vi "createWriterQueue.vi"(0 "QueueName":string, 2 "WriterEndPointName":string, 5 "error in":errorcluster, 6 "ReaderEndPointName":string, 8 "Remote application Name":string) -> (19 "error out":errorcluster)   [LabVIEW 2013]
doc: "Used as a mechanism to have queue notification across process boundaries using network streams. No need to define a shared variable. Put the vi outside of the loop in parallel, and define a named queue to communicate through the link.\n\nRemote application Name - Remote application process instance name that tells the writer where to send the data \nReaderEndPointName - Used to build up the application context indicating the endpoint to stream data. Make sure that this matches both sides of the link.\nQueueName - Named queue to be used within the process.\nWriterEndPointName - Application process instance name that indicates where the data stream is sourced from"
uses:
  control/payloadData.ctl
  control/cmdQueueWriterRef.ctl
  Global/GlobalStop.vi
  <resource>/objmgr/ni.dex.rc
panel:
  out "Main Loop":i32
  out "writerURL":string
  out "Application:Name":string
  out "errorLoop":i32
  out "readerURL":string
  out "Acquire loop":i32
  out "queue OP":T1
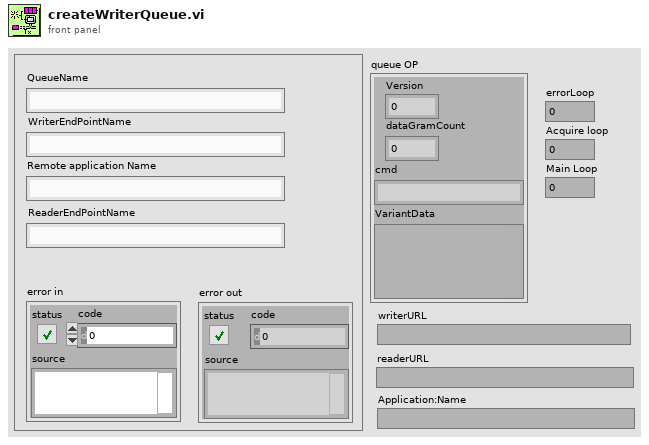
[diagram p1: front panel]
types:
  T1 = typedef "payloadData.ctl" = cluster{"Version":u32, "dataGramCount":i32, "cmd":string, "VariantData":variant}
  T2 = enum32{"invalid app kind", "Development System", "Run Time System", "Student Edition", "Embedded LabVIEW", "Evaluation", "Custom"}
  T3 = typedef "cmdQueueWriterRef.ctl" = cluster{"cmd":string, "msgQueue":refnum<queue>, "writerEndPoint":refnum<k21>}
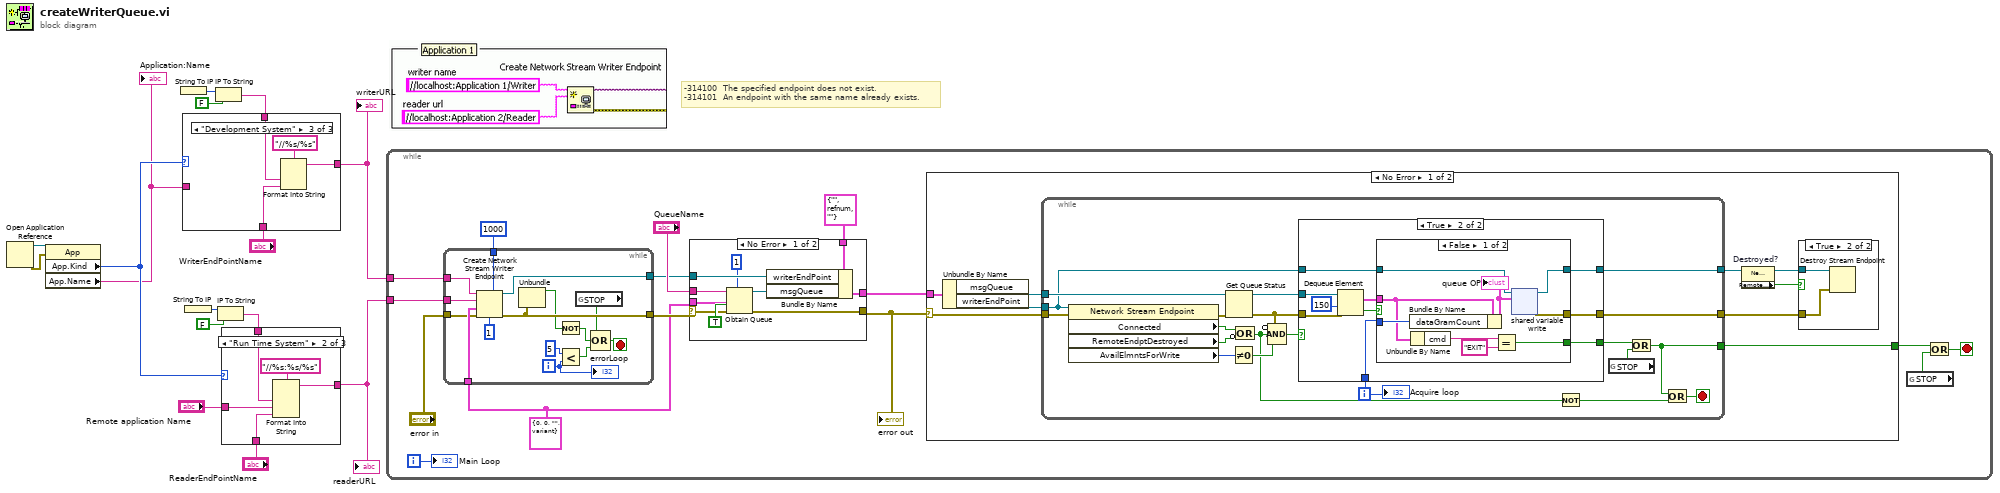
[diagram p0: block diagram]
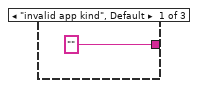
[diagram p2: hidden frame]
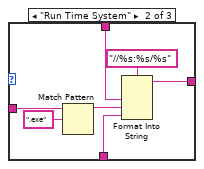
[diagram p3: hidden frame]
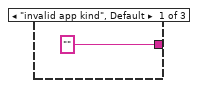
[diagram p4: hidden frame]
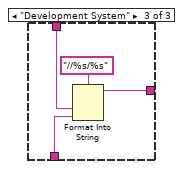
[diagram p5: hidden frame]
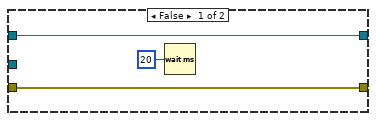
[diagram p7: hidden frame]
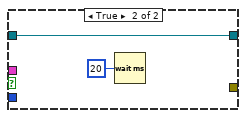
[diagram p8: hidden frame]
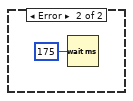
[diagram p9: hidden frame]
diagram:
  # "-314100 \tThe specified endpoint does not exist. \n-314101 \tAn endpoint with the same name already exists."
  n1 = Open Application Reference() -> (0:w14:errorcluster, 3:w15:refnum<vi>)  [unwired: 4 in]
  n2 = property class="App"(reference=w15, error in=w14) -> ("App.Kind"=w4:T2, "App.Name"=w2:string)  [unwired: 2 out]
  "Application:Name" <- w2
  n3 = String To IP() -> (0:w12:u32)  [unwired: 1 in]
  n4 = String To IP() -> (0:w8:u32)  [unwired: 1 in]
  n5 = IP To String(1:FALSE ("dot notation? (F)"), 2:w12) -> (0:w9:string)
  n6 = case shown="\"Development System\"" w4 {
    tunnel: w9 -> [_ w22 w26]
    tunnel: ["" w21 w25] -> w1
    tunnel: "WriterEndPointName" -> [_ w20 w24]
    tunnel: w2 -> [_ w18 _]
    frame "invalid app kind", Default {
    }
    frame "Run Time System" {
      n7 = Match Pattern(string=w18, regular expression=".exe") -> (before substring=w19:string)  [unwired: 1 in, 3 out]
      n8 = Format Into String(format string="//%s:%s/%s", w22, w19, w20) -> (resulting string=w21:string)  [unwired: 2 in, 1 out]
    }
    frame "Development System" {
      n9 = Format Into String(format string="//%s/%s", w26, w24) -> (resulting string=w25:string)  [unwired: 2 in, 1 out]
    }
  }
  "writerURL" <- w1
  n10 = IP To String(1:FALSE ("dot notation? (F)"), 2:w8) -> (0:w6:string)
  n11 = case shown="\"Run Time System\"" w4 {
    tunnel: w6 -> [_ w32 w36]
    tunnel: ["" w31 w35] -> w11
    tunnel: "ReaderEndPointName" -> [_ w30 w34]
    tunnel: "Remote application Name" -> [_ w29 _]
    frame "invalid app kind", Default {
    }
    frame "Run Time System" {
      n12 = Format Into String(format string="//%s:%s/%s", w32, w29, w30) -> (resulting string=w31:string)  [unwired: 2 in, 1 out]
    }
    frame "Development System" {
      n13 = Format Into String(format string="//%s/%s", w36, w34) -> (resulting string=w35:string)  [unwired: 2 in, 1 out]
    }
  }
  "readerURL" <- w11
  n14 = while {
    tunnel: w11 -> [w44]
    tunnel: w1 -> [w43]
    i -> [w40]
    stop <- w39 stop-if-true
    w50 = T1 {"Version"=0, "dataGramCount"=0, "cmd"="", "VariantData"=variant} ("Data")
    n15 = while {
      tunnel: w50 -> [w122]
      tunnel: [w111] -> w42
      tunnel: w44 -> [w114]
      tunnel: "error in" -> [w121]
      tunnel: [w112] -> w52
      tunnel: 1000 ("timeout in ms (-1)") -> [w115]
      tunnel: w43 -> [w113]
      i -> [w120]
      stop <- w116 stop-if-true
      n16 = Create Network Stream Writer Endpoint(5:w115, 7:1 ("writer buffer size"), 8:w121, 9:w122, 10:w114, 11:w113) -> (0:w112:errorcluster, 3:w111:refnum<k21>)  [unwired: 1 in]
      n17 = Unbundle(w112) -> ("status"=w110:bool)  [unwired: 2 out]
      n18 = Not(x=w110) -> (.not. x?=w117:bool)
      n19 = Less?(x=5, y=w120) -> (x < y?=w118:bool)
      n20 = global read "GlobalStop.vi" "STOP"() -> (w109:bool)
      n21 = Compound Arithmetic op=OR(w109, w117, w118) -> (w116:bool)
      "errorLoop" <- w120
    }
    n22 = case shown="No Error" w52 {
      selector: w52 -> [w129 w134]
      tunnel: [w133 _] -> w47
      tunnel: [w132 w134] -> w48
      tunnel: "QueueName" -> [w131 _]
      tunnel: w50 -> [w128 _]
      tunnel: w42 -> [w127 _]
      tunnel: T3 {"cmd"="", "msgQueue"=refnum, "writerEndPoint"=""} ("msgRef") -> [w124 _]
      frame No Error {
        n23 = Obtain Queue(max queue size (-1, unlimited)=1 ("writer buffer size"), name (unnamed)=w131, element data type=w128, create if not found? (T)=TRUE, error in (no error)=w129) -> (queue out=w126:refnum<queue>, error out=w132:errorcluster)  [unwired: 1 out]
        n24 = Bundle By Name(cluster=w124, "writerEndPoint"=w127, "msgQueue"=w126) -> (w133:T3)
      }
      frame Error {
      }
    }
    "error out" <- w48
    n25 = case shown="No Error" w48 {
      selector: w48 -> [w61 _]
      tunnel: w47 -> [w58 _]
      tunnel: [w57 _] -> w41
      frame No Error {
        n26 = Unbundle By Name(w58) -> ("msgQueue"=w59:refnum<queue>, "writerEndPoint"=w60:refnum<k21>)
        n27 = while {
          tunnel: w61 -> [w83]
          tunnel: w60 -> [w78]
          tunnel: w59 -> [w82]
          tunnel: [w72] -> w53
          tunnel: [w66] -> w57
          tunnel: [w69] -> w54
          i -> [w71]
          stop <- w68 stop-if-true
          n28 = property class="Network Stream Endpoint"(reference=w78, error in=w83) -> (error out=w70:errorcluster, "Connected"=w81:bool, "RemoteEndptDestroyed"=w75:bool, "AvailElmntsForWrite"=w80:i32)  [unwired: 1 out]
          n29 = Get Queue Status(queue=w82, error in (no error)=w70) -> (queue out=w79:refnum<queue>, error out=w73:errorcluster)  [unwired: 1 in, 6 out]
          n30 = Not Equal To 0?(x=w80) -> (x != 0?=w77:bool)
          n31 = Compound Arithmetic op=OR(w81, invert w75) -> (w74:bool)
          n32 = Compound Arithmetic op=AND(invert w73, w74, w77) -> (w76:bool)
          n33 = case shown="True" w76 {
            tunnel: w79 -> [_ w94]
            tunnel: w78 -> [w84 w92]
            tunnel: w73 -> [w86 w91]
            tunnel: [w86 w87] -> w72
            tunnel: w71 -> [_ w90]
            tunnel: [_ w89] -> w65
            tunnel: [w84 w88] -> w69
            frame False {
              n34 = Wait (ms)(milliseconds to wait=u32 20) -> ()  [unwired: 1 out]
            }
            frame True {
              n35 = Dequeue Element(queue=w94, timeout in ms (-1)=150, error in (no error)=w91) -> (element=w93:T1, timed out?=w96:bool)  [unwired: 2 out]
              n36 = case shown="False" w96 {
                tunnel: w93 -> [w102 _]
                tunnel: w92 -> [w105 w106]
                tunnel: w90 -> [w104 _]
                tunnel: [w99 _] -> w89
                tunnel: [w98 w106] -> w88
                tunnel: [w97 _] -> w87
                frame False {
                  n37 = Bundle By Name(cluster=w102, "dataGramCount"=w104) -> (w103:T1)
                  "queue OP" <- w103
                  n38 = Unbundle By Name(w102) -> ("cmd"=w101:string)
                  n39 = Equal?(x=w101, y="EXIT") -> (x = y?=w99:bool)
                  n40 = shared-variable-write(w105, w103) -> (w98:refnum<k21>, w97:errorcluster)  [unwired: 2 in, 1 out]
                }
                frame True {
                  n41 = Wait (ms)(milliseconds to wait=u32 20) -> ()  [unwired: 1 out]
                }
              }
            }
          }
          n42 = Not(x=w74) -> (.not. x?=w67:bool)
          n43 = global read "GlobalStop.vi" "STOP"() -> (w64:bool)
          n44 = Or(x=w65, y=w64) -> (x .or. y?=w66:bool)
          n45 = Or(x=w66, y=w67) -> (x .or. y?=w68:bool)
          "Acquire loop" <- w71
        }
        n46 = property on="Destroyed?" class="Network Stream Endpoint"(reference=w54) -> (reference out=w55:refnum<k21>, "RemoteEndptDestroyed"=w56:bool)  [unwired: 1 in, 1 out]
        n47 = case shown="True" w56 {
          tunnel: w55 -> [_ w63]
          tunnel: w53 -> [_ w62]
          frame False {
          }
          frame True {
            n48 = Destroy Stream Endpoint(8:w62, 11:w63) -> ()  [unwired: 1 out]
          }
        }
      }
      frame Error {
        n49 = Wait (ms)(milliseconds to wait=u32 175) -> ()  [unwired: 1 out]
      }
    }
    n50 = global read "GlobalStop.vi" "STOP"() -> (w38:bool)
    n51 = Or(x=w41, y=w38) -> (x .or. y?=w39:bool)
    "Main Loop" <- w40
  }
